vi "保存用户信息.vi"(8 "error in (no error)":errorcluster caption="错误输入（无错误）", 11 "用户信息":T1(array[cluster])) -> (0 "error out":errorcluster caption="错误输出")   [LabVIEW 2016, in "Alarm interface.lvlib" / "wxpusher.lvlib"]
uses:
  wxpusher.lvlib
  <vilib>/Utility/sysdir.llb/System Directory Type.ctl
  <vilib>/Utility/config.llb/Write Key (String).vi
  <vilib>/Utility/config.llb/NI_LVConfig.lvlib
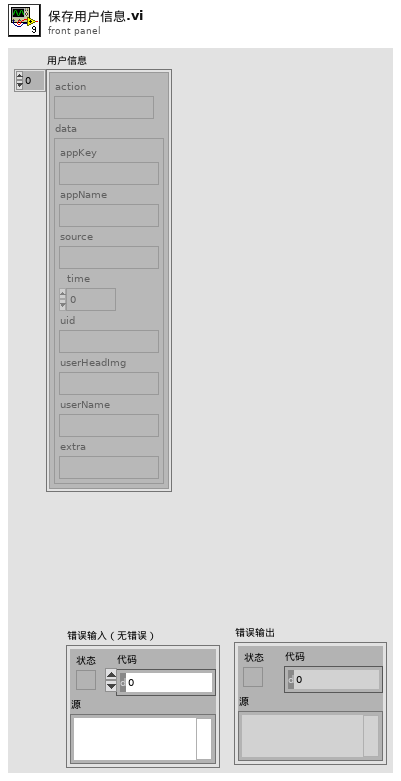
[diagram p1: front panel]
types:
  T1 = cluster{"action":string, "data":cluster{"appKey":string, "appName":string, "source":string, "time":u64, "uid":string, "userHeadImg":string, "userName":string, "extra":string}}[]
  T2 = typedef "System Directory Type.ctl" = i32
  T3 = typedef "NI_LVConfig.lvlib/Config Data RefNum.ctl" = refnum<k1>
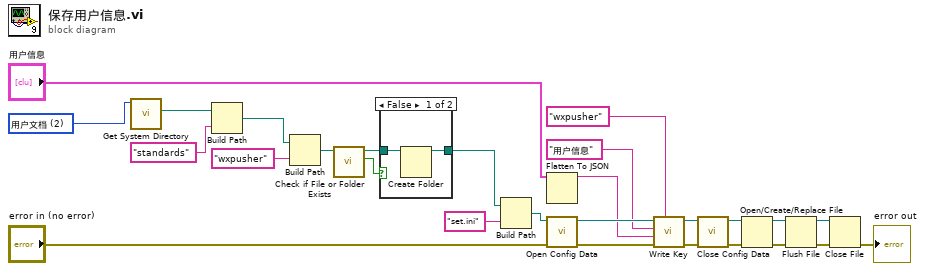
[diagram p0: block diagram]
diagram:
  w18 = T2 2 items=["用户目录"=0, "用户桌面"=1, "用户文档"=2, "用户应用程序数据"=3, "用户设置"=4, "用户临时目录"=5, "公共文档"=6, "公共应用程序数据"=7, "公共设置"=8, "公共缓存"=13, "系统核心库"=9, "系统安装库"=10, "应用程序文件"=11, "启动盘根目录"=12] ("system directory type")
  n1 = call <vilib>:"Get System Directory.vi"("system directory type"=w18) -> ("system directory"=w19:path)  [unwired: 10 in]
  n2 = Build Path(base path=w19, name or relative path="standards" ("名称或相对路径")) -> (appended path=w16:path)
  n3 = Build Path(base path=w16, name or relative path="wxpusher" ("名称或相对路径")) -> (appended path=w23:path)
  n4 = call <vilib>:"Check if File or Folder Exists.vi"("path"=w23) -> ("file or folder exists?"=w22:bool, "dup path"=w21:path)  [unwired: 8 in, 1 out]
  n5 = case shown="False" w22 {
    tunnel: w21 -> [w29 w30]
    tunnel: [w28 w30] -> w20
    frame False {
      n6 = Create Folder(path (use dialog)=w29) -> (created path=w28:path)  [unwired: 2 in, 2 out]
    }
    frame True {
    }
  }
  n7 = Build Path(base path=w20, name or relative path="set.ini" ("名称或相对路径")) -> (appended path=w26:path)
  n8 = Flatten To JSON(anything="用户信息") -> (JSON string=w9:string)  [unwired: 2 in, 1 out]
  n9 = call <vilib>:"Open Config Data.vi"("error in (no error)"="error in (no error)", "configuration file path"=w26) -> ("error out"=w13:errorcluster, "refnum"=w14:T3)  [unwired: 7 in, 1 out]
  n10 = call-poly <vilib>:"Write Key.vi"("section"="wxpusher", "error in (no error)"=w13, "value"=w9, "key"="用户信息", "refnum"=w14) -> ("error out"=w11:errorcluster, "refnum out"=w12:T3)  [unwired: 4 in, 1 out]
  n11 = call <vilib>:"Close Config Data.vi"("error in (no error)"=w11, "refnum"=w12) -> ("error out"=w2:errorcluster, "file path"=w3:path)  [unwired: 8 in]
  n12 = Open/Create/Replace File(file path (use dialog)=w3, error in=w2) -> (refnum out=w7:refnum<file>, error out=w5:errorcluster)  [unwired: 4 in, 1 out]
  n13 = Flush File(refnum=w7, error in=w5) -> (refnum out=w6:refnum<file>, error out=w4:errorcluster)
  n14 = Close File(refnum=w6, error in=w4) -> (error out=→"error out":errorcluster)  [unwired: 1 out]
